vi "AIARG-UWKWT-Calibrate-Driver.vi"() -> ()   [LabVIEW 2017]
uses:
  <vilib>/Analysis/Matrix/Datatypes/RealMatrix.ctl
  <vilib>/Analysis/6fits.llb/Curve Fitting Criteria.ctl
  <vilib>/Analysis/baseanly.llb/Mean (DBL).vi
  <vilib>/ULx/Create Channel.llb/ULx Create Channel (AI-Voltage-Basic).vi
  <vilib>/ULx/Timing.llb/ULx Timing (Sample Clock).vi
  <vilib>/ULx/Read.llb/ULx Read (Analog Wfm 1Chan NSamp).vi
  <vilib>/Utility/file.llb/Write Delimited Spreadsheet (DBL).vi
  <vilib>/Analysis/Matrix/Numeric/Conversions/Array To Matrix - RA.vi
  <vilib>/Analysis/NI_AALBase.lvlib
  <vilib>/Analysis/Matrix/NI_Matrix.lvlib
  <vilib>/Analysis/NI_AALPro.lvlib
panel:
  out "Rolling Moment R-Squared":dbl
  out "Rolling Moment Intercept":dbl
  out "Rolling Moment Slope":dbl
  out "S.F. R-Squared":dbl
  out "S.F. Intercept":dbl
  out "S.F. Slope":dbl
  out "P.M. R-Squared":dbl
  out "P.M. Intercept":dbl
  out "P.M. Slope":dbl
  out "n R-Squared":dbl
  out "n Intercept":dbl
  out "n Slope":dbl
  out "Axial R-Squared":dbl
  out "Axial Intercept":dbl
  out "Axial Slope":dbl
  out "Normal R-Squared":dbl
  out "Normal Intercept":dbl
  out "Normal Slope":dbl
  out "Main Graph Intercept":dbl
  out "Main Graph R-Squared":dbl
  out "Main Graph Slope":dbl
  out "Axial":cluster{"Weight":dbl[], "Voltage(Axial)":dbl[]}(graph)
  out "Rolling Moment":cluster{"Weight":dbl[], "Voltage(R.M.) ":dbl[]}(graph)
  out "S.F.":cluster{"Weight":dbl[], "Voltage(S.F.)":dbl[]}(graph)
  out "P.M.":cluster{"Weight":dbl[], "Voltage(P.M.)":dbl[]}(graph)
  out "n":cluster{"Weight":dbl[], "Voltage(n)":dbl[]}(graph)
  out "Normal":cluster{"Weight":dbl[], "Voltage(Normal)":dbl[]}(graph)
  out "Main Graph":cluster{"Weight":dbl[], "Main Voltage":dbl[]}[](graph)
  out "Matrix Path Indicator":path
  in  "Record Matrix Path":path
  in  "Final Matrix":T1
  out "R.M. Sample Waveform":dbl[](graph)
  out "S.F. Sample Waveform":dbl[](graph)
  out "P.M. Sample Waveform":dbl[](graph)
  out "n Sample Waveform":dbl[](graph)
  out "Axial Force Sample Waveform":dbl[](graph)
  out "Normal Force Sample Waveform":dbl[](graph)
  out "Main Voltage":dbl[](array[numeric])
  out "Current Main Channel Calibration":string
  in  "Main Channel":string(combo)
  in  "Rolling Moment Physical Channel":refnum<k21>
  in  "S.F. Physical Channel":refnum<k21>
  in  "P.M. Physical Channel":refnum<k21>
  in  "n Physical Channel":refnum<k21>
  in  "Normal Force Physical Channel":refnum<k21>
  in  "minimum value":dbl=-5.0
  in  "maximum value":dbl=5.0
  in  "samples per channel":i32=100
  in  "sample mode":i32(ring) items=["FiniteSamples", "ContinuousSamples"]
  in  "rate":dbl=5000.0
  in  "Axial Force Physical Channel":refnum<k21>
  out "Voltage(R.M.)":dbl[](array[numeric])
  out "Voltage(S.F.)":dbl[](array[numeric])
  out "Voltage(P.M.)":dbl[](array[numeric])
  out "Voltage(n)":dbl[](array[numeric])
  out "Voltage(Normal)":dbl[](array[numeric])
  in  "Sample Button":bool
  in  "Add Weight":bool
  in  "Weight to be added":dbl
  out "Voltage(Axial)":dbl[](array[numeric])
  out "Weight":dbl[](array[numeric])
  in  "Clear Table":bool
  # "Channel and Sampling Selection"
  # "Interaction Plots\n\nPlots ALL SIX voltages,"
  # "Voltages from EACH Channel\nRecords data from all six channels for each sample cycle. Each number represents the mean of all values from one sample cycle recorded by one channel."
  # "Sample Waveform Graphs\n\nPlots all the data points onto a waveform graph in one sample Cycle, to see the range of noises and determine any bias in data."
  # "Final Matrix\nThe final matrix that records the data from calibration and overwrites itself every time one calibration cycle is performed."
  # "Weight"
  # "Normal Force"
  # "Axial Force"
  # "n"
  # "P.M."
  # "S.F."
  # "Rolling Moment"
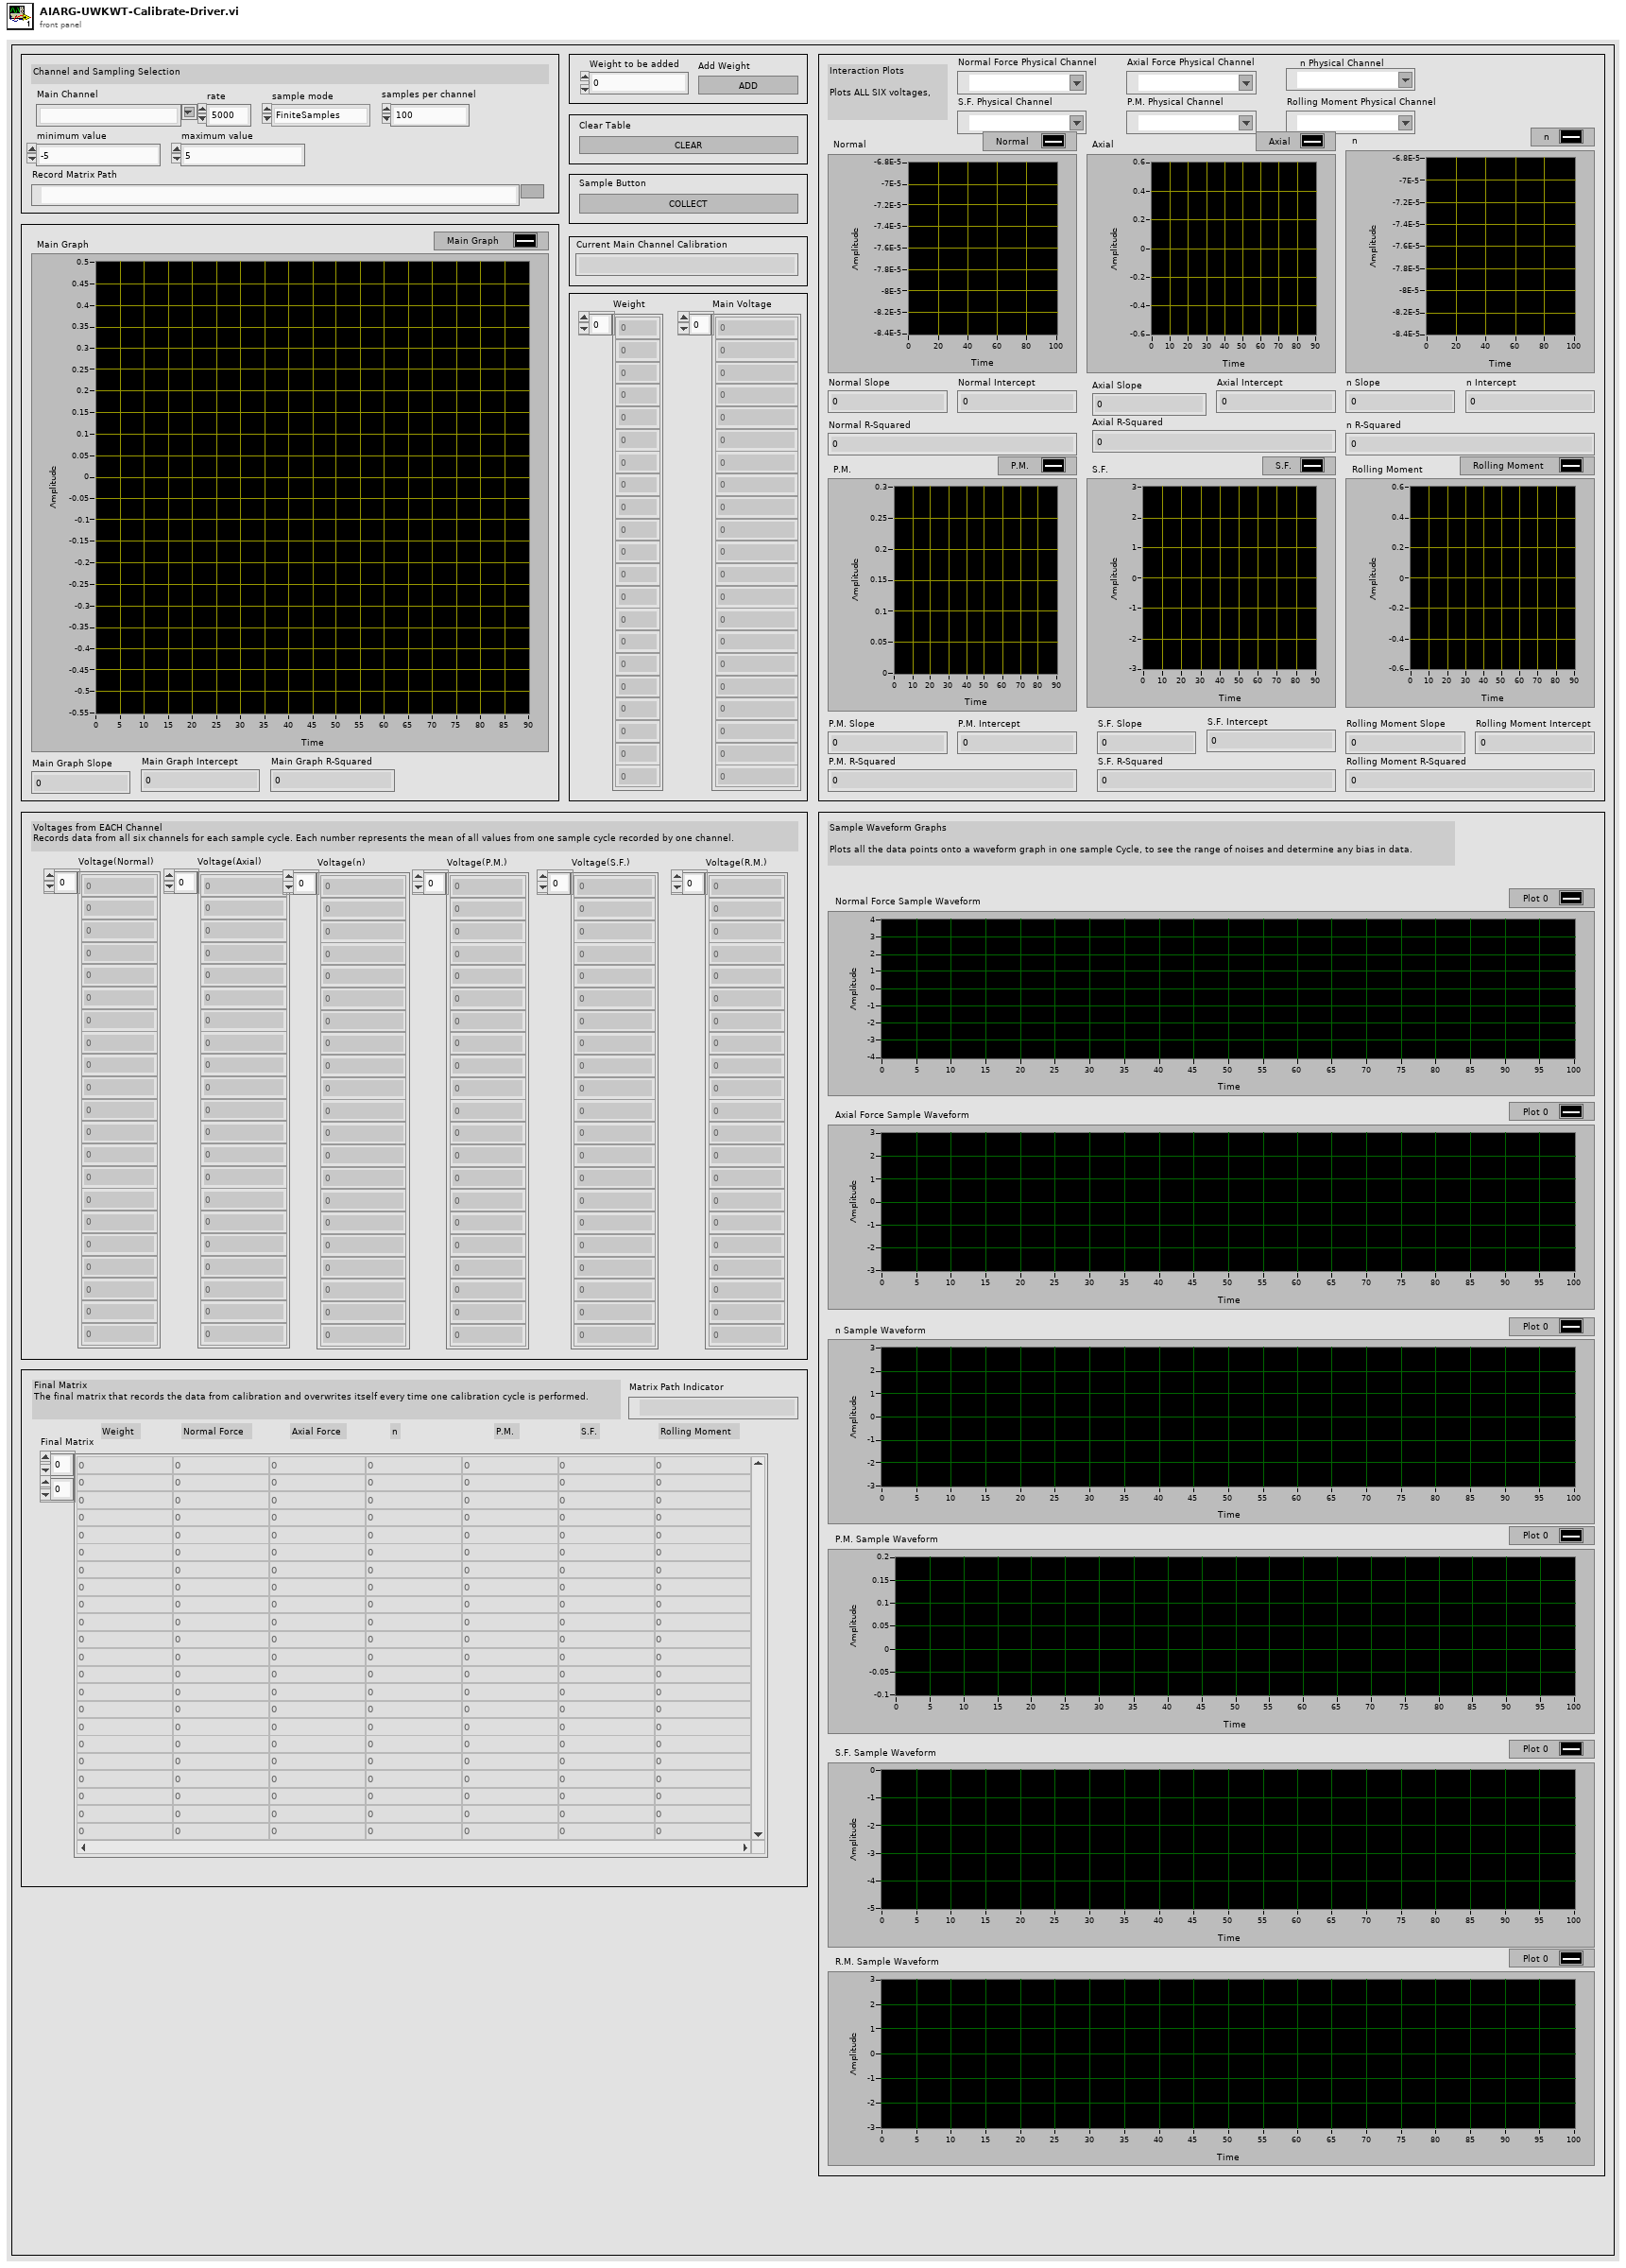
[diagram p1: front panel]
types:
  T1 = typedef "NI_Matrix.lvlib/RealMatrix.ctl" = dbl[][]
  T2 = typedef "NI_AALPro.lvlib/Curve Fitting Criteria.ctl" = u16
  T3 = cluster{"Weight":dbl[], "Best Linear Fit":dbl[]}[]
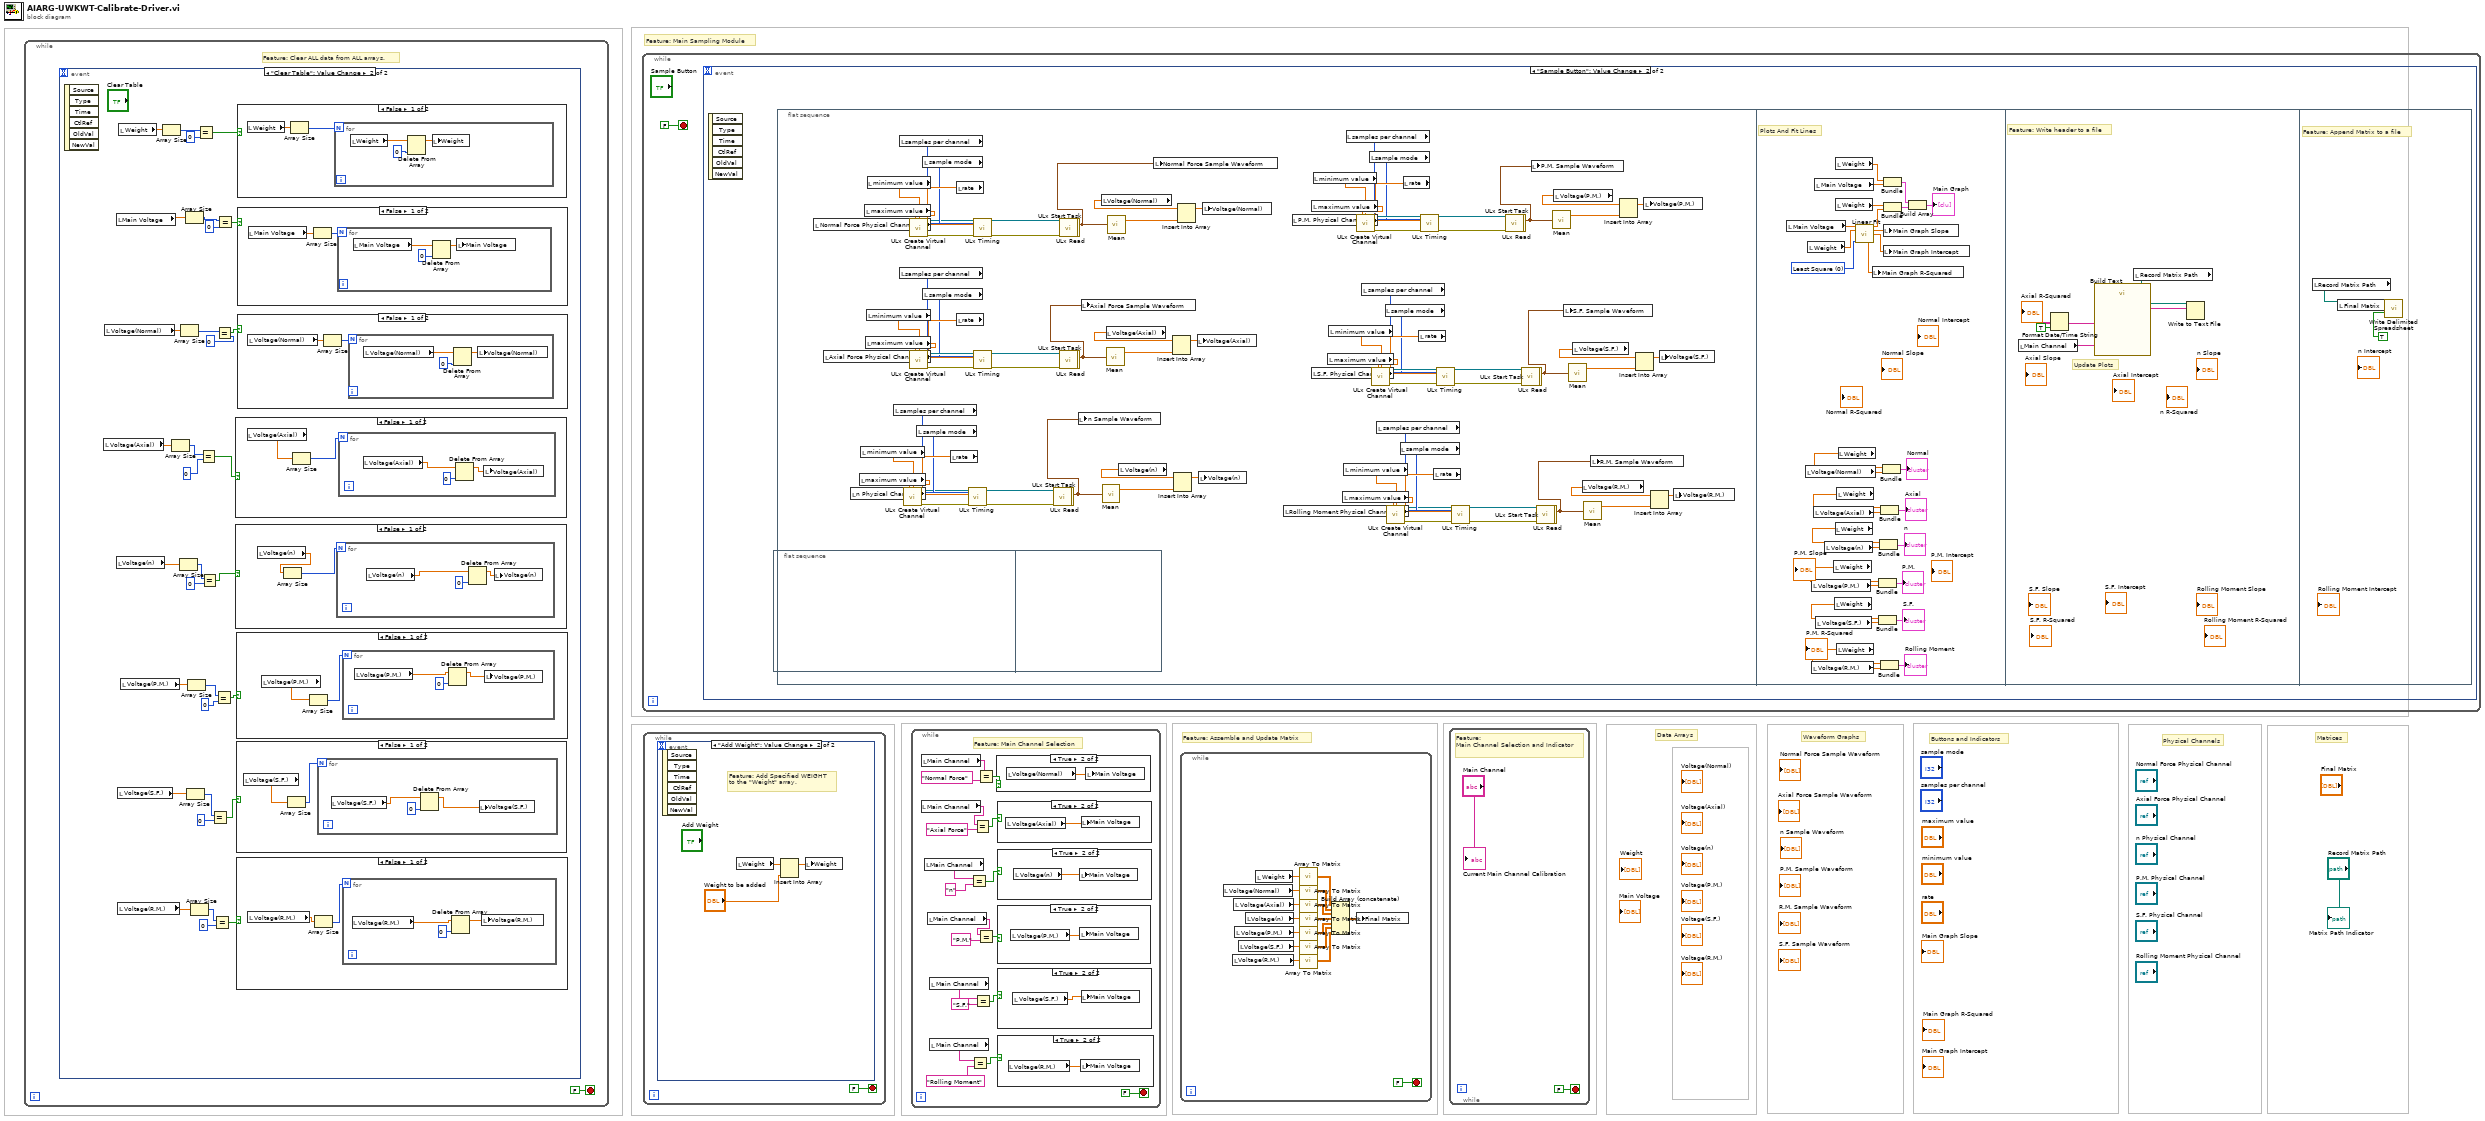
[diagram p0: block diagram]
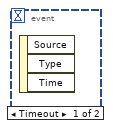
[diagram p8: hidden frame]
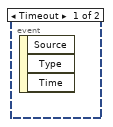
[diagram p17: hidden frame]
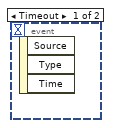
[diagram p18: hidden frame]
diagram:
  # "Matrices"
  # "Feature: Assemble and Update Matrix"
  # "Waveform Graphs"
  # "Physical Channels"
  # "Feature: Main Sampling Module"
  # "Data Arrays"
  # "Buttons and Indicators"
  n1 = while {
    stop <- FALSE stop-if-true
    # "Feature: Clear ALL data from ALL arrays."
    n2 = event shown="[1] \"Clear Table\": Value Change" {
      selector: _ -> [_ _]
      dyn-events: _ -> [_ _]
      timeout: _ -> [_ _]
      event Timeout {
        n3 = event-data() -> ()  [unwired: 1 in, 3 out]
      }
      event "Clear Table": Value Change {
        n4 = event-data() -> ()  [unwired: 1 in, 6 out]
        n5 = local read "Voltage(Axial)"() -> (w21:dbl[])
        n6 = local read "Voltage(Normal)"() -> (w24:dbl[])
        n7 = local read "Main Voltage"() -> (w30:dbl[])
        n8 = local read "Voltage(n)"() -> (w18:dbl[])
        n9 = local read "Voltage(S.F.)"() -> (w10:dbl[])
        n10 = local read "Voltage(R.M.)"() -> (w6:dbl[])
        n11 = local read "Weight"() -> (w31:dbl[])
        n12 = local read "Voltage(P.M.)"() -> (w13:dbl[])
        n13 = Array Size(array=w31) -> (size(s)=w34:i32)
        n14 = Array Size(array=w21) -> (size(s)=w22:i32)
        n15 = Array Size(array=w18) -> (size(s)=w17:i32)
        n16 = Array Size(array=w24) -> (size(s)=w25:i32)
        n17 = Array Size(array=w30) -> (size(s)=w29:i32)
        n18 = Array Size(array=w10) -> (size(s)=w9:i32)
        n19 = Array Size(array=w13) -> (size(s)=w14:i32)
        n20 = Array Size(array=w6) -> (size(s)=w5:i32)
        n21 = Equal?(x=w34, y=0) -> (x = y?=w32:bool)
        n22 = Equal?(x=w22, y=0) -> (x = y?=w19:bool)
        n23 = Equal?(x=w17, y=0) -> (x = y?=w15:bool)
        n24 = Equal?(x=w9, y=0) -> (x = y?=w7:bool)
        n25 = Equal?(x=w5, y=0) -> (x = y?=w4:bool)
        n26 = Equal?(x=w14, y=0) -> (x = y?=w11:bool)
        n27 = Equal?(x=w25, y=0) -> (x = y?=w26:bool)
        n28 = Equal?(x=w29, y=0) -> (x = y?=w27:bool)
        n29 = case shown="False" w19 {
          frame False {
            n30 = local read "Voltage(Axial)"() -> (w56:dbl[])
            n31 = Array Size(array=w56) -> (size(s)=w55:i32)
            n32 = for {
              N: w55 -> [_]
              n33 = local read "Voltage(Axial)"() -> (w59:dbl[])
              n34 = Delete From Array(array=w59, index=0) -> (array with subset deleted=w57:dbl[])  [unwired: 1 in, 1 out]
              n35 = local write "Voltage(Axial)"(w57) -> ()
            }
          }
          frame True {
          }
        }
        n36 = case shown="False" w15 {
          frame False {
            n37 = local read "Voltage(n)"() -> (w51:dbl[])
            n38 = Array Size(array=w51) -> (size(s)=w50:i32)
            n39 = for {
              N: w50 -> [_]
              n40 = local read "Voltage(n)"() -> (w54:dbl[])
              n41 = Delete From Array(array=w54, index=0) -> (array with subset deleted=w52:dbl[])  [unwired: 1 in, 1 out]
              n42 = local write "Voltage(n)"(w52) -> ()
            }
          }
          frame True {
          }
        }
        n43 = case shown="False" w11 {
          frame False {
            n44 = local read "Voltage(P.M.)"() -> (w46:dbl[])
            n45 = Array Size(array=w46) -> (size(s)=w45:i32)
            n46 = for {
              N: w45 -> [_]
              n47 = local read "Voltage(P.M.)"() -> (w49:dbl[])
              n48 = Delete From Array(array=w49, index=0) -> (array with subset deleted=w47:dbl[])  [unwired: 1 in, 1 out]
              n49 = local write "Voltage(P.M.)"(w47) -> ()
            }
          }
          frame True {
          }
        }
        n50 = case shown="False" w7 {
          frame False {
            n51 = local read "Voltage(S.F.)"() -> (w41:dbl[])
            n52 = Array Size(array=w41) -> (size(s)=w40:i32)
            n53 = for {
              N: w40 -> [_]
              n54 = local read "Voltage(S.F.)"() -> (w44:dbl[])
              n55 = Delete From Array(array=w44, index=0) -> (array with subset deleted=w43:dbl[])  [unwired: 1 in, 1 out]
              n56 = local write "Voltage(S.F.)"(w43) -> ()
            }
          }
          frame True {
          }
        }
        n57 = case shown="False" w4 {
          frame False {
            n58 = local read "Voltage(R.M.)"() -> (w35:dbl[])
            n59 = Array Size(array=w35) -> (size(s)=w36:i32)
            n60 = for {
              N: w36 -> [_]
              n61 = local read "Voltage(R.M.)"() -> (w39:dbl[])
              n62 = Delete From Array(array=w39, index=0) -> (array with subset deleted=w37:dbl[])  [unwired: 1 in, 1 out]
              n63 = local write "Voltage(R.M.)"(w37) -> ()
            }
          }
          frame True {
          }
        }
        n64 = case shown="False" w26 {
          frame False {
            n65 = local read "Voltage(Normal)"() -> (w61:dbl[])
            n66 = Array Size(array=w61) -> (size(s)=w60:i32)
            n67 = for {
              N: w60 -> [_]
              n68 = local read "Voltage(Normal)"() -> (w64:dbl[])
              n69 = Delete From Array(array=w64, index=0) -> (array with subset deleted=w63:dbl[])  [unwired: 1 in, 1 out]
              n70 = local write "Voltage(Normal)"(w63) -> ()
            }
          }
          frame True {
          }
        }
        n71 = case shown="False" w32 {
          frame False {
            n72 = local read "Weight"() -> (w71:dbl[])
            n73 = Array Size(array=w71) -> (size(s)=w70:i32)
            n74 = for {
              N: w70 -> [_]
              n75 = local read "Weight"() -> (w73:dbl[])
              n76 = Delete From Array(array=w73, index=0) -> (array with subset deleted=w72:dbl[])  [unwired: 1 in, 1 out]
              n77 = local write "Weight"(w72) -> ()
            }
          }
          frame True {
          }
        }
        n78 = case shown="False" w27 {
          frame False {
            n79 = local read "Main Voltage"() -> (w66:dbl[])
            n80 = Array Size(array=w66) -> (size(s)=w65:i32)
            n81 = for {
              N: w65 -> [_]
              n82 = local read "Main Voltage"() -> (w68:dbl[])
              n83 = Delete From Array(array=w68, index=0) -> (array with subset deleted=w69:dbl[])  [unwired: 1 in, 1 out]
              n84 = local write "Main Voltage"(w69) -> ()
            }
          }
          frame True {
          }
        }
      }
    }
  }
  n85 = while {
    stop <- FALSE stop-if-true
    n86 = event shown="[1] \"Sample Button\": Value Change" {
      selector: _ -> [_ _]
      dyn-events: _ -> [_ _]
      timeout: _ -> [_ _]
      event Timeout {
        n87 = event-data() -> ()  [unwired: 1 in, 3 out]
      }
      event "Sample Button": Value Change {
        n88 = event-data() -> ()  [unwired: 1 in, 6 out]
        n89 = flat-sequence {
          frame #0 {
          }
          frame #1 {
          }
        }
        n90 = flat-sequence {
          frame #0 {
            n91 = local read "Normal Force Physical Channel"() -> (w156:refnum<k21>)
            n92 = local read "Axial Force Physical Channel"() -> (w157:refnum<k21>)
            n93 = local read "n Physical Channel"() -> (w141:refnum<k21>)
            n94 = local read "maximum value"() -> (w137:dbl)
            n95 = local read "minimum value"() -> (w136:dbl)
            n96 = local read "maximum value"() -> (w154:dbl)
            n97 = local read "maximum value"() -> (w161:dbl)
            n98 = local read "minimum value"() -> (w168:dbl)
            n99 = local read "minimum value"() -> (w155:dbl)
            n100 = local read "samples per channel"() -> (w139:i32)
            n101 = local read "samples per channel"() -> (w150:i32)
            n102 = local read "samples per channel"() -> (w158:i32)
            n103 = call-poly <vilib>:"ULx Create Virtual Channel.vi"("maximum value"=w137, "minimum value"=w136, "physical channels"=w141) -> ("task out"=w127:refnum<k24>, "error out"=w128:errorcluster)  [unwired: 11 in]
            n104 = call-poly <vilib>:"ULx Create Virtual Channel.vi"("maximum value"=w154, "minimum value"=w155, "physical channels"=w156) -> ("task out"=w149:refnum<k24>, "error out"=w153:errorcluster)  [unwired: 11 in]
            n105 = call-poly <vilib>:"ULx Create Virtual Channel.vi"("maximum value"=w161, "minimum value"=w168, "physical channels"=w157) -> ("task out"=w162:refnum<k24>, "error out"=w167:errorcluster)  [unwired: 11 in]
            n106 = local read "sample mode"() -> (w138:i32)
            n107 = local read "sample mode"() -> (w151:i32)
            n108 = local read "sample mode"() -> (w159:i32)
            n109 = local read "rate"() -> (w140:dbl)
            n110 = local read "rate"() -> (w152:dbl)
            n111 = local read "rate"() -> (w160:dbl)
            n112 = call-poly <vilib>:"ULx Timing.vi"("task in"=w127, "sample mode"=w138, "samples per channel"=w139, "rate"=w140, "error in"=w128) -> ("task out"=w130:refnum<k24>, "error out"=w129:errorcluster)  [unwired: 9 in]
            n113 = call-poly <vilib>:"ULx Timing.vi"("task in"=w149, "sample mode"=w151, "samples per channel"=w150, "rate"=w152, "error in"=w153) -> ("task out"=w148:refnum<k24>, "error out"=w147:errorcluster)  [unwired: 9 in]
            n114 = call-poly <vilib>:"ULx Timing.vi"("task in"=w162, "sample mode"=w159, "samples per channel"=w158, "rate"=w160, "error in"=w167) -> ("task out"=w163:refnum<k24>, "error out"=w166:errorcluster)  [unwired: 9 in]
            n115 = call <vilib>:"ULx Start Task.vi"("task in"=w130, "error in"=w129) -> ("task out"=w132:refnum<k24>, "error out"=w131:errorcluster)  [unwired: 12 in]
            n116 = call-poly <vilib>:"ULx Read.vi"("task in"=w132, "error in"=w131) -> ("data"=w79:waveform(dbl))  [unwired: 11 in, 2 out]
            n117 = call <vilib>:"ULx Start Task.vi"("task in"=w148, "error in"=w147) -> ("task out"=w146:refnum<k24>, "error out"=w145:errorcluster)  [unwired: 12 in]
            n118 = call <vilib>:"ULx Start Task.vi"("task in"=w163, "error in"=w166) -> ("task out"=w164:refnum<k24>, "error out"=w165:errorcluster)  [unwired: 12 in]
            n119 = call-poly <vilib>:"ULx Read.vi"("task in"=w146, "error in"=w145) -> ("data"=w81:waveform(dbl))  [unwired: 11 in, 2 out]
            n120 = call-poly <vilib>:"ULx Read.vi"("task in"=w164, "error in"=w165) -> ("data"=w80:waveform(dbl))  [unwired: 11 in, 2 out]
            n121 = local write "n Sample Waveform"(w79) -> ()
            n122 = local write "Axial Force Sample Waveform"(w80) -> ()
            n123 = local read "Voltage(Normal)"() -> (w143:dbl[])
            n124 = call-poly <vilib>:"Mean.vi"("X"=w79) -> ("mean"=w133:dbl)  [unwired: 1 out]
            n125 = local read "Voltage(Axial)"() -> (w170:dbl[])
            n126 = call-poly <vilib>:"Mean.vi"("X"=w80) -> ("mean"=w169:dbl)  [unwired: 1 out]
            n127 = call-poly <vilib>:"Mean.vi"("X"=w81) -> ("mean"=w144:dbl)  [unwired: 1 out]
            n128 = local read "Voltage(n)"() -> (w135:dbl[])
            n129 = local write "Normal Force Sample Waveform"(w81) -> ()
            n130 = Insert Into Array(array=w170, new element=w169) -> (w171:dbl[])  [unwired: 1 in]
            n131 = Insert Into Array(array=w135, new element=w133) -> (w134:dbl[])  [unwired: 1 in]
            n132 = Insert Into Array(array=w143, new element=w144) -> (w142:dbl[])  [unwired: 1 in]
            n133 = local write "Voltage(Axial)"(w171) -> ()
            n134 = local write "Voltage(n)"(w134) -> ()
            n135 = local write "Voltage(Normal)"(w142) -> ()
            n136 = local read "Rolling Moment Physical Channel"() -> (w100:refnum<k21>)
            n137 = local read "P.M. Physical Channel"() -> (w126:refnum<k21>)
            n138 = local read "S.F. Physical Channel"() -> (w101:refnum<k21>)
            n139 = local read "maximum value"() -> (w125:dbl)
            n140 = local read "minimum value"() -> (w124:dbl)
            n141 = local read "maximum value"() -> (w98:dbl)
            n142 = local read "minimum value"() -> (w99:dbl)
            n143 = local read "maximum value"() -> (w86:dbl)
            n144 = local read "minimum value"() -> (w87:dbl)
            n145 = local read "samples per channel"() -> (w116:i32)
            n146 = call-poly <vilib>:"ULx Create Virtual Channel.vi"("maximum value"=w125, "minimum value"=w124, "physical channels"=w126) -> ("task out"=w123:refnum<k24>, "error out"=w114:errorcluster)  [unwired: 11 in]
            n147 = local read "samples per channel"() -> (w95:i32)
            n148 = local read "sample mode"() -> (w115:i32)
            n149 = call-poly <vilib>:"ULx Create Virtual Channel.vi"("maximum value"=w98, "minimum value"=w99, "physical channels"=w101) -> ("task out"=w97:refnum<k24>, "error out"=w96:errorcluster)  [unwired: 11 in]
            n150 = local read "samples per channel"() -> (w89:i32)
            n151 = local read "sample mode"() -> (w94:i32)
            n152 = call-poly <vilib>:"ULx Create Virtual Channel.vi"("maximum value"=w86, "minimum value"=w87, "physical channels"=w100) -> ("task out"=w85:refnum<k24>, "error out"=w84:errorcluster)  [unwired: 11 in]
            n153 = local read "sample mode"() -> (w88:i32)
            n154 = local read "rate"() -> (w122:dbl)
            n155 = local read "rate"() -> (w121:dbl)
            n156 = call-poly <vilib>:"ULx Timing.vi"("task in"=w123, "sample mode"=w115, "samples per channel"=w116, "rate"=w122, "error in"=w114) -> ("task out"=w113:refnum<k24>, "error out"=w112:errorcluster)  [unwired: 9 in]
            n157 = local read "rate"() -> (w120:dbl)
            n158 = call-poly <vilib>:"ULx Timing.vi"("task in"=w97, "sample mode"=w94, "samples per channel"=w95, "rate"=w121, "error in"=w96) -> ("task out"=w93:refnum<k24>, "error out"=w92:errorcluster)  [unwired: 9 in]
            n159 = call-poly <vilib>:"ULx Timing.vi"("task in"=w85, "sample mode"=w88, "samples per channel"=w89, "rate"=w120, "error in"=w84) -> ("task out"=w83:refnum<k24>, "error out"=w82:errorcluster)  [unwired: 9 in]
            n160 = call <vilib>:"ULx Start Task.vi"("task in"=w113, "error in"=w112) -> ("task out"=w111:refnum<k24>, "error out"=w110:errorcluster)  [unwired: 12 in]
            n161 = call-poly <vilib>:"ULx Read.vi"("task in"=w111, "error in"=w110) -> ("data"=w77:waveform(dbl))  [unwired: 11 in, 2 out]
            n162 = call <vilib>:"ULx Start Task.vi"("task in"=w93, "error in"=w92) -> ("task out"=w91:refnum<k24>, "error out"=w90:errorcluster)  [unwired: 12 in]
            n163 = call-poly <vilib>:"ULx Read.vi"("task in"=w91, "error in"=w90) -> ("data"=w76:waveform(dbl))  [unwired: 11 in, 2 out]
            n164 = local write "P.M. Sample Waveform"(w77) -> ()
            n165 = call <vilib>:"ULx Start Task.vi"("task in"=w83, "error in"=w82) -> ("task out"=w106:refnum<k24>, "error out"=w105:errorcluster)  [unwired: 12 in]
            n166 = call-poly <vilib>:"ULx Read.vi"("task in"=w106, "error in"=w105) -> ("data"=w78:waveform(dbl))  [unwired: 11 in, 2 out]
            n167 = call-poly <vilib>:"Mean.vi"("X"=w77) -> ("mean"=w119:dbl)  [unwired: 1 out]
            n168 = local read "Voltage(P.M.)"() -> (w118:dbl[])
            n169 = local write "S.F. Sample Waveform"(w76) -> ()
            n170 = call-poly <vilib>:"Mean.vi"("X"=w76) -> ("mean"=w104:dbl)  [unwired: 1 out]
            n171 = local read "Voltage(S.F.)"() -> (w103:dbl[])
            n172 = local read "Voltage(R.M.)"() -> (w108:dbl[])
            n173 = call-poly <vilib>:"Mean.vi"("X"=w78) -> ("mean"=w107:dbl)  [unwired: 1 out]
            n174 = local write "R.M. Sample Waveform"(w78) -> ()
            n175 = Insert Into Array(array=w118, new element=w119) -> (w117:dbl[])  [unwired: 1 in]
            n176 = Insert Into Array(array=w103, new element=w104) -> (w102:dbl[])  [unwired: 1 in]
            n177 = local write "Voltage(P.M.)"(w117) -> ()
            n178 = Insert Into Array(array=w108, new element=w107) -> (w109:dbl[])  [unwired: 1 in]
            n179 = local write "Voltage(S.F.)"(w102) -> ()
            n180 = local write "Voltage(R.M.)"(w109) -> ()
          }
          frame #1 {
            w176 = T2 0 items=["Least Square", "Least Absolute Residual", "Bisquare"] ("method")
            # "Plots And Fit Lines"
            n181 = local read "Main Voltage"() -> (w180:dbl[])
            n182 = local read "Voltage(Normal)"() -> (w200:dbl[])
            n183 = local read "Weight"() -> (w181:dbl[])
            n184 = local read "Voltage(P.M.)"() -> (w192:dbl[])
            n185 = local read "Voltage(R.M.)"() -> (w186:dbl[])
            n186 = local read "Voltage(Axial)"() -> (w197:dbl[])
            n187 = local read "Main Voltage"() -> (w202:dbl[])
            n188 = local read "Voltage(S.F.)"() -> (w189:dbl[])
            n189 = local read "Voltage(n)"() -> (w195:dbl[])
            n190 = local read "Weight"() -> (w193:dbl[])
            n191 = local read "Weight"() -> (w190:dbl[])
            n192 = local read "Weight"() -> (w196:dbl[])
            n193 = local read "Weight"() -> (w175:dbl[])
            n194 = local read "Weight"() -> (w173:dbl[])
            n195 = local read "Weight"() -> (w187:dbl[])
            n196 = local read "Weight"() -> (w198:dbl[])
            n197 = local read "Weight"() -> (w201:dbl[])
            n198 = call <vilib>:"Linear Fit.vi"("Y"=w180, "X"=w181, "method"=w176) -> ("Best Linear Fit"=w172:dbl[], "slope"=w179:dbl, "intercept"=w178:dbl, "residue"=w177:dbl)  [unwired: 8 in, 1 out]
            n199 = local write "Main Graph R-Squared"(w177) -> ()
            n200 = Bundle("Weight"=w193, "Voltage(P.M.)"=w192) -> (→"P.M.":cluster{"Weight":dbl[], "Voltage(P.M.)":dbl[]})  [unwired: 1 in]
            n201 = Bundle("Weight"=w190, "Voltage(S.F.)"=w189) -> (→"S.F.":cluster{"Weight":dbl[], "Voltage(S.F.)":dbl[]})  [unwired: 1 in]
            n202 = Bundle("Weight"=w196, "Voltage(n)"=w195) -> (→"n":cluster{"Weight":dbl[], "Voltage(n)":dbl[]})  [unwired: 1 in]
            n203 = Bundle("Weight"=w187, "Voltage(R.M.)"=w186) -> (→"Rolling Moment":cluster{"Weight":dbl[], "Voltage(R.M.) ":dbl[]})  [unwired: 1 in]
            n204 = Bundle("Weight"=w198, "Voltage(Axial)"=w197) -> (→"Axial":cluster{"Weight":dbl[], "Voltage(Axial)":dbl[]})  [unwired: 1 in]
            n205 = Bundle("Weight"=w201, "Voltage(Normal)"=w200) -> (→"Normal":cluster{"Weight":dbl[], "Voltage(Normal)":dbl[]})  [unwired: 1 in]
            n206 = Bundle("Weight"=w175, "Main Voltage"=w202) -> (w182:cluster{"Weight":dbl[], "Main Voltage":dbl[]})  [unwired: 1 in]
            n207 = Bundle("Weight"=w173, "Best Linear Fit"=w172) -> (w174:cluster{"Weight":dbl[], "Best Linear Fit":dbl[]})  [unwired: 1 in]
            n208 = local write "Main Graph Slope"(w179) -> ()
            n209 = local write "Main Graph Intercept"(w178) -> ()
            n210 = Build Array(w182, w174) -> (→"Main Graph":T3)
          }
          frame #2 {
            # "Feature: Write header to a file"
            # "Update Plots"
            n211 = local read "Main Channel"() -> (w204:string)
            n212 = Format Date/Time String(UTC format=TRUE) -> (date/time string=w206:string)  [unwired: 2 in]
            n213 = call "Build Text"("date"=w206, "mainchannel"=w204) -> ("Result"=w205:string)  [unwired: 12 in, 1 out]
            n214 = local read "Record Matrix Path"() -> (w207:path)
            n215 = Write to Text File(file (use dialog)=w207, text=w205) -> ()  [unwired: 2 in, 3 out]
          }
          frame #3 {
            # "Feature: Append Matrix to a file"
            n216 = local read "Record Matrix Path"() -> (w209:path)
            n217 = local read "Final Matrix"() -> (w210:T1)
            n218 = call-poly <vilib>:"Write Delimited Spreadsheet.vi"("file path (dialog if empty)"=w209, "2D data"=w210, "append to file? (new file:F)"=TRUE) -> ()  [unwired: 11 in, 2 out]
          }
        }
      }
    }
  }
  n219 = while {
    stop <- FALSE stop-if-true
    n220 = event shown="[1] \"Add Weight\": Value Change" {
      selector: _ -> [_ _]
      dyn-events: _ -> [_ _]
      timeout: _ -> [_ _]
      event Timeout {
        n221 = event-data() -> ()  [unwired: 1 in, 3 out]
      }
      event "Add Weight": Value Change {
        # "Feature: Add Specified WEIGHT\nto the \"Weight\" array."
        n222 = event-data() -> ()  [unwired: 1 in, 6 out]
        n223 = local read "Weight"() -> (w213:dbl[])
        n224 = Insert Into Array(array=w213, new element="Weight to be added") -> (w212:dbl[])  [unwired: 1 in]
        n225 = local write "Weight"(w212) -> ()
      }
    }
  }
  n226 = while {
    stop <- FALSE stop-if-true
    # "Feature: Main Channel Selection"
    n227 = local read "Main Channel"() -> (w229:string)
    n228 = local read "Main Channel"() -> (w232:string)
    n229 = local read "Main Channel"() -> (w225:string)
    n230 = local read "Main Channel"() -> (w223:string)
    n231 = local read "Main Channel"() -> (w221:string)
    n232 = local read "Main Channel"() -> (w219:string)
    n233 = Equal?(x=w225, y="n") -> (x = y?=w226:bool)
    n234 = Equal?(x=w219, y="Rolling Moment") -> (x = y?=w220:bool)
    n235 = Equal?(x=w229, y="Axial Force") -> (x = y?=w228:bool)
    n236 = Equal?(x=w221, y="S.F.") -> (x = y?=w222:bool)
    n237 = Equal?(x=w232, y="Normal Force") -> (x = y?=w230:bool)
    n238 = Equal?(x=w223, y="P.M.") -> (x = y?=w224:bool)
    n239 = case shown="True" w230 {
      frame False {
      }
      frame True {
        n240 = local read "Voltage(Normal)"() -> (w239:dbl[])
        n241 = local write "Main Voltage"(w239) -> ()
      }
    }
    n242 = case shown="True" w228 {
      frame False {
      }
      frame True {
        n243 = local read "Voltage(Axial)"() -> (w238:dbl[])
        n244 = local write "Main Voltage"(w238) -> ()
      }
    }
    n245 = case shown="True" w226 {
      frame False {
      }
      frame True {
        n246 = local read "Voltage(n)"() -> (w237:dbl[])
        n247 = local write "Main Voltage"(w237) -> ()
      }
    }
    n248 = case shown="True" w224 {
      frame False {
      }
      frame True {
        n249 = local read "Voltage(P.M.)"() -> (w236:dbl[])
        n250 = local write "Main Voltage"(w236) -> ()
      }
    }
    n251 = case shown="True" w222 {
      frame False {
      }
      frame True {
        n252 = local read "Voltage(S.F.)"() -> (w235:dbl[])
        n253 = local write "Main Voltage"(w235) -> ()
      }
    }
    n254 = case shown="True" w220 {
      frame False {
      }
      frame True {
        n255 = local read "Voltage(R.M.)"() -> (w234:dbl[])
        n256 = local write "Main Voltage"(w234) -> ()
      }
    }
  }
  n257 = while {
    stop <- FALSE stop-if-true
    n258 = local read "Voltage(Normal)"() -> (w253:dbl[])
    n259 = local read "Voltage(R.M.)"() -> (w246:dbl[])
    n260 = local read "Voltage(Axial)"() -> (w250:dbl[])
    n261 = local read "Voltage(P.M.)"() -> (w248:dbl[])
    n262 = local read "Voltage(S.F.)"() -> (w247:dbl[])
    n263 = local read "Voltage(n)"() -> (w249:dbl[])
    n264 = local read "Weight"() -> (w251:dbl[])
    n265 = call-poly <vilib>:"Array To Matrix.vi"("Real 1D Array"=w251) -> ("Real Matrix (Column Vector)"=w252:T1)
    n266 = call-poly <vilib>:"Array To Matrix.vi"("Real 1D Array"=w253) -> ("Real Matrix (Column Vector)"=w254:T1)
    n267 = call-poly <vilib>:"Array To Matrix.vi"("Real 1D Array"=w250) -> ("Real Matrix (Column Vector)"=w245:T1)
    n268 = call-poly <vilib>:"Array To Matrix.vi"("Real 1D Array"=w249) -> ("Real Matrix (Column Vector)"=w244:T1)
    n269 = call-poly <vilib>:"Array To Matrix.vi"("Real 1D Array"=w248) -> ("Real Matrix (Column Vector)"=w243:T1)
    n270 = call-poly <vilib>:"Array To Matrix.vi"("Real 1D Array"=w247) -> ("Real Matrix (Column Vector)"=w242:T1)
    n271 = call-poly <vilib>:"Array To Matrix.vi"("Real 1D Array"=w246) -> ("Real Matrix (Column Vector)"=w241:T1)
    n272 = Build Array (concatenate)(w252, w254, w245, w244, w243, w242, w241) -> (w240:T1)
    n273 = local write "Final Matrix"(w240) -> ()
  }
  n274 = while {
    stop <- FALSE stop-if-true
    # "Feature:\nMain Channel Selection and Indicator"
    "Current Main Channel Calibration" <- "Main Channel"
  }
  "Matrix Path Indicator" <- "Record Matrix Path"
